vi "Host - TCP - Engine.vi"() -> ()   [LabVIEW 2017]
uses:
  TCP Engine/SubVIs/Read File.ctl
  TCP Engine/Controls/RT- Queue States.ctl
  TCP Engine/TCP/TCP - Signals.ctl
  TCP Engine/TCP/TCP - Signal Names.ctl
  Controls/Control - Testscreen.ctl
  RT/Test Execution/Test - Step Result.ctl
  Controls/Test details.ctl
  TCP Engine/TCP/TCP - Driver Control.ctl
  Variable/Global 1.vi
  TCP Engine/TCP/TCP - Test Settings.ctl
  RT/Controls/RT- Get Set.ctl
panel:
  out "Log Path 2":path
  out "Log Path":path
  out "Waveform Chart":u32(graph)
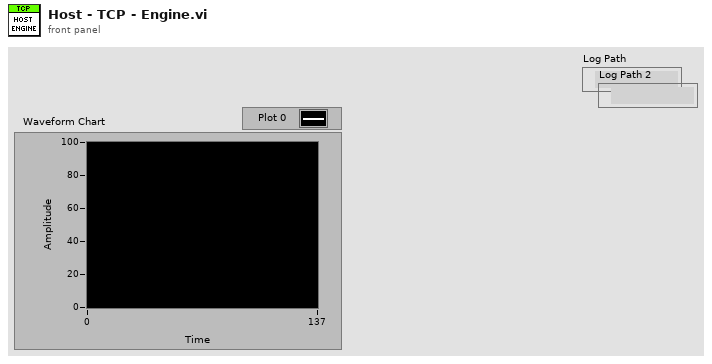
[diagram p1: front panel]
types:
  T1 = typedef "RT- Queue States.ctl" = enum16{"Initialize", "Enqueue", "Enqueue Priority", "Dequeue", "Flush", "Destroy"}
  T2 = typedef "Read File.ctl" = enum16{"Fetch XML", "Open", "Read", "Write", "Close"}
  T3 = typedef "TCP - Test Settings.ctl" = cluster{"Sequence File":string, "Iteration":i32}
  T4 = typedef "TCP - Signals.ctl" = cluster{"Signal":T5, "Value":bool, "Data":variant}
  T5 = typedef "TCP - Signal Names.ctl" = enum16{"Test Running", "Update Sensor Data", "Start Test", "Test Started", "Sequence Complete", "Seuence Aborted", "Abort Test", "Test Settings Updated", "Log Path", "Update Manual Values", "Start Aux Logging", "Aux Log Started", "Stop Aux Logging", "Aux Log Stopped", "Set Dyno Config", "Get PID Values", "Reset Emergency", "Copy Log File", "Download Files", "Send Test Details"}
  T6 = typedef "Control - Testscreen.ctl" = enum16{"No Event", "Init", "Download Files", "Test Running", "Update Test Results", "Machine Unhealthy", "Autotest Started", "Test Aborted", "Sequence Complete", "Update Sensor Data", "Log File Available", "Machine Mode", "Aux Logging Started", "Aux File Saved", "Get PID Values", "View Report", "Exit", "Wait", "Abort", "Copy Log File", "Send Test Details"}
  T7 = typedef "Test - Step Result.ctl" = cluster{"Step Name":string, "Value":dbl, "Success ?":bool, "Stop Seq ?":bool, "Abort":bool, "Sr.No":i32}
  T8 = typedef "RT- Get Set.ctl" = enum16{"Reset", "Get", "Set"}
  T9 = typedef "Test details.ctl" = cluster{"Furnace":string, "Material":string, "Angle":string, "ID":string, "Flowrate":string, "Test Name":string, "Tested By":string}
  T10 = typedef "TCP - Driver Control.ctl" = enum16{"Test Settings", "Boolean Commands", "Test Results", "Send Test Details"}
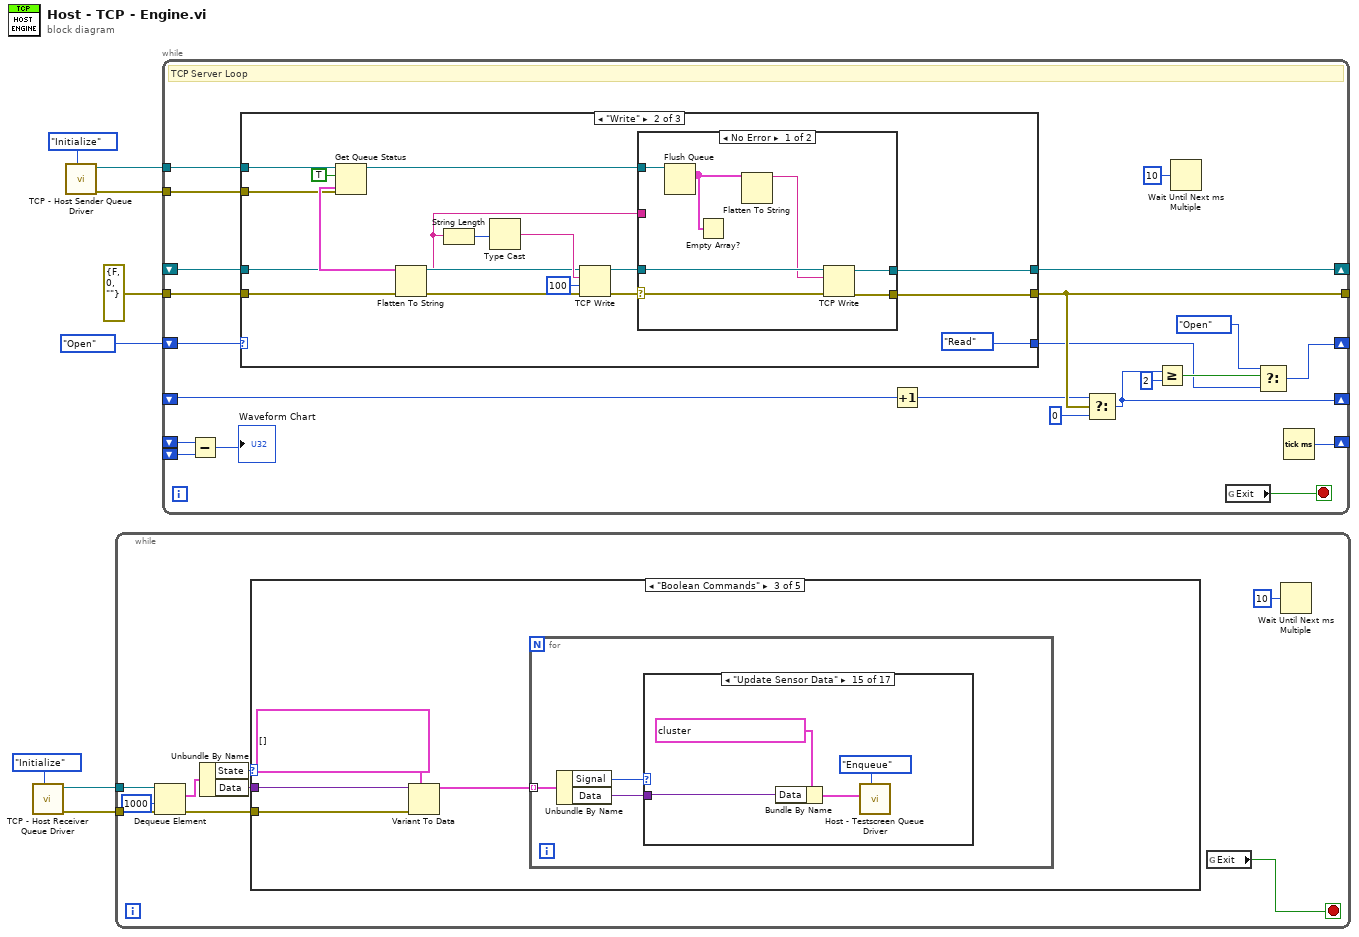
[diagram p0: block diagram]
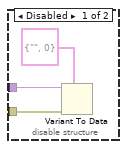
[diagram p3: hidden frame]
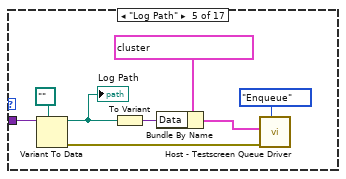
[diagram p9: hidden frame]
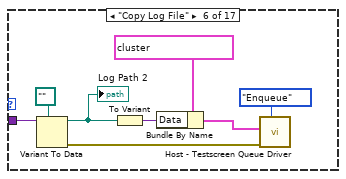
[diagram p10: hidden frame]
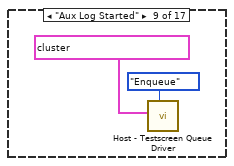
[diagram p13: hidden frame]
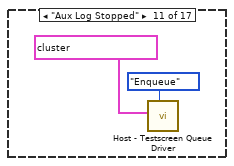
[diagram p15: hidden frame]
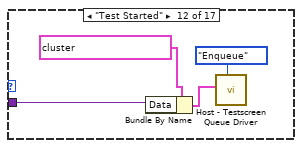
[diagram p16: hidden frame]
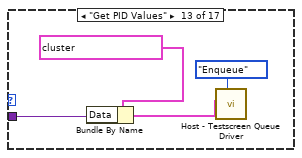
[diagram p17: hidden frame]
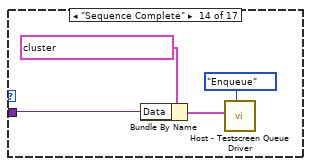
[diagram p18: hidden frame]
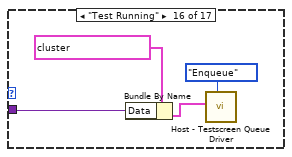
[diagram p19: hidden frame]
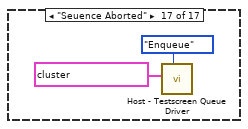
[diagram p20: hidden frame]
diagram:
  n1 = call "TCP - Host Receiver Queue Driver.vi"("Cases"=RT-_Queue_States."Initialize") -> ("error out"=w5:errorcluster, "queue out"=w6:refnum<queue>)  [unwired: 8 in, 1 out]
  n2 = call "TCP - Host Sender Queue Driver.vi"("Cases"=RT-_Queue_States."Initialize") -> ("error out"=w1:errorcluster, "queue out"=w2:refnum<queue>)  [unwired: 8 in, 1 out]
  n3 = while {
    tunnel: w6 -> [w16]
    tunnel: w5 -> [w17]
    stop <- w9 stop-if-true
    n4 = Dequeue Element(queue=w16, timeout in ms (-1)=1000, error in (no error)=w17) -> (element=w14:cluster{"Data":variant, "State":T10}, error out=w15:errorcluster)  [unwired: 2 out]
    n5 = Unbundle By Name(w14) -> ("State"=w12:T10, "Data"=w11:variant)
    n6 = case shown="\"Boolean Commands\"" w12 {
      tunnel: w15 -> [w19 _ w25 w80 w97]
      tunnel: w11 -> [w18 _ w26 w81 w98]
      frame "Test Settings" {
        n7 = disable-structure shown="Enabled" {
          disable-tunnel: w19 -> [w22 _]
          disable-tunnel: w18 -> [w21 _]
          frame Disabled {
            n8 = Variant To Data(error in=w22, type=T3 {"Sequence File"="", "Iteration"=0}, Variant=w21) -> ()  [unwired: 2 out]
          }
          frame Enabled {
          }
        }
      }
      frame Default {
      }
      frame "Boolean Commands" {
        n9 = Variant To Data(error in=w25, type=T4[] [], Variant=w26) -> (data=w23:T4[])  [unwired: 1 out]
        n10 = for {
          tunnel: w23 -> [w29] mode=indexing
          n11 = Unbundle By Name(w29) -> ("Signal"=w28:T5, "Data"=w27:variant)
          n12 = case shown="\"Update Sensor Data\"" w28 {
            tunnel: w27 -> [_ _ _ _ w37 w45 _ _ _ _ _ w52 w55 w60 w64 w68 _]
            frame "Start Test", Default {
            }
            frame "Abort Test" {
            }
            frame "Test Settings Updated" {
            }
            frame "Set Dyno Config" {
            }
            frame "Log Path" {
              n13 = Variant To Data(type=path "", Variant=w37) -> (data=w32:path, error out=w34:errorcluster)  [unwired: 1 in]
              "Log Path" <- w32
              n14 = To Variant(anything=w32) -> (Variant=w31:variant)
              n15 = Bundle By Name(cluster=cluster{"Data":variant, "Enum":T6} {"Data"=variant, "Enum"=enum."Log File Available"} ("Element In"), "Data"=w31) -> (w30:cluster{"Data":variant, "Enum":T6})
              n16 = call "Host - Testscreen Queue Driver.vi"("Cases"=RT-_Queue_States."Enqueue", "error in (no error)"=w34, "Element In"=w30) -> ()  [unwired: 6 in, 3 out]
            }
            frame "Copy Log File" {
              n17 = Variant To Data(type=path "", Variant=w45) -> (data=w40:path, error out=w42:errorcluster)  [unwired: 1 in]
              "Log Path 2" <- w40
              n18 = To Variant(anything=w40) -> (Variant=w39:variant)
              n19 = Bundle By Name(cluster=cluster{"Data":variant, "Enum":T6} {"Data"=variant, "Enum"=enum."Copy Log File"} ("Element In"), "Data"=w39) -> (w38:cluster{"Data":variant, "Enum":T6})
              n20 = call "Host - Testscreen Queue Driver.vi"("Cases"=RT-_Queue_States."Enqueue", "error in (no error)"=w42, "Element In"=w38) -> ()  [unwired: 6 in, 3 out]
            }
            frame "Update Manual Values" {
            }
            frame "Start Aux Logging" {
            }
            frame "Aux Log Started" {
              n21 = call "Host - Testscreen Queue Driver.vi"("Cases"=RT-_Queue_States."Enqueue", "Element In"=cluster{"Data":variant, "Enum":T6} {"Data"=variant, "Enum"=enum."Aux Logging Started"}) -> ()  [unwired: 7 in, 3 out]
            }
            frame "Stop Aux Logging" {
            }
            frame "Aux Log Stopped" {
              n22 = call "Host - Testscreen Queue Driver.vi"("Cases"=RT-_Queue_States."Enqueue", "Element In"=cluster{"Data":variant, "Enum":T6} {"Data"=variant, "Enum"=enum."Aux File Saved"}) -> ()  [unwired: 7 in, 3 out]
            }
            frame "Test Started" {
              n23 = Bundle By Name(cluster=cluster{"Data":variant, "Enum":T6} {"Data"=variant, "Enum"=enum."Autotest Started"} ("Element In"), "Data"=w52) -> (w50:cluster{"Data":variant, "Enum":T6})
              n24 = call "Host - Testscreen Queue Driver.vi"("Cases"=RT-_Queue_States."Enqueue", "Element In"=w50) -> ()  [unwired: 7 in, 3 out]
            }
            frame "Get PID Values" {
              n25 = Bundle By Name(cluster=cluster{"Data":variant, "Enum":T6} {"Data"=variant, "Enum"=enum."Get PID Values"} ("Element In"), "Data"=w55) -> (w54:cluster{"Data":variant, "Enum":T6})
              n26 = call "Host - Testscreen Queue Driver.vi"("Cases"=RT-_Queue_States."Enqueue", "Element In"=w54) -> ()  [unwired: 7 in, 3 out]
            }
            frame "Sequence Complete" {
              n27 = Bundle By Name(cluster=cluster{"Data":variant, "Enum":T6} {"Data"=variant, "Enum"=enum."Sequence Complete"} ("Element In"), "Data"=w60) -> (w58:cluster{"Data":variant, "Enum":T6})
              n28 = call "Host - Testscreen Queue Driver.vi"("Cases"=RT-_Queue_States."Enqueue", "Element In"=w58) -> ()  [unwired: 7 in, 3 out]
            }
            frame "Update Sensor Data" {
              n29 = Bundle By Name(cluster=cluster{"Data":variant, "Enum":T6} {"Data"=variant, "Enum"=enum."Update Sensor Data"} ("Element In"), "Data"=w64) -> (w62:cluster{"Data":variant, "Enum":T6})
              n30 = call "Host - Testscreen Queue Driver.vi"("Cases"=RT-_Queue_States."Enqueue", "Element In"=w62) -> ()  [unwired: 7 in, 3 out]
            }
            frame "Test Running" {
              n31 = Bundle By Name(cluster=cluster{"Data":variant, "Enum":T6} {"Data"=variant, "Enum"=enum."Test Running"} ("Element In"), "Data"=w68) -> (w66:cluster{"Data":variant, "Enum":T6})
              n32 = call "Host - Testscreen Queue Driver.vi"("Cases"=RT-_Queue_States."Enqueue", "Element In"=w66) -> ()  [unwired: 7 in, 3 out]
            }
            frame "Seuence Aborted" {
              n33 = call "Host - Testscreen Queue Driver.vi"("Cases"=RT-_Queue_States."Enqueue", "Element In"=cluster{"Data":variant, "Enum":T6} {"Data"=variant, "Enum"=enum."Test Aborted"}) -> ()  [unwired: 7 in, 3 out]
            }
          }
        }
      }
      frame "Test Results" {
        n34 = Variant To Data(error in=w80, type=T7 {"Step Name"="", "Value"=0.0, "Success ?"=TRUE, "Stop Seq ?"=TRUE, "Abort"=TRUE, "Sr.No"=0} ("element"), Variant=w81) -> (data=w77:T7, error out=w76:errorcluster)
        n35 = disable-structure shown="Enabled" {
          disable-tunnel: w77 -> [w84 w88]
          disable-tunnel: w76 -> [w83 w87]
          disable-tunnel: [w82 w87] -> w75
          disable-tunnel: [_ w86] -> w73
          frame Disabled {
            n36 = call "Test - FGV - Test Results.vi"("Get/Set"=RT-_Get_Set."Set", "error in (no error)"=w83, "Step Result"=w84) -> ("error out"=w82:errorcluster)  [unwired: 7 in, 1 out]
          }
          frame Enabled {
            n37 = To Variant(anything=w88) -> (Variant=w86:variant)
          }
        }
        n38 = Bundle By Name(cluster=cluster{"Data":variant, "Enum":T6} {"Data"=variant, "Enum"=enum."Update Test Results"} ("Element In"), "Data"=w73) -> (w72:cluster{"Data":variant, "Enum":T6})
        n39 = call "Host - Testscreen Queue Driver.vi"("Cases"=RT-_Queue_States."Enqueue", "error in (no error)"=w75, "Element In"=w72) -> ()  [unwired: 6 in, 3 out]
      }
      frame "Send Test Details" {
        (unwired) T7 {"Step Name"="", "Value"=0.0, "Success ?"=TRUE, "Stop Seq ?"=TRUE, "Abort"=TRUE, "Sr.No"=0} ("element")
        n40 = Variant To Data(error in=w97, type=T9 {"Furnace"="Furnace A", "Material"="Coke", "Angle"="Multi Angle", "ID"="Trajectory 9", "Flowrate"="Flow", "Test Name"="Coke Burn", "Tested By"="Anirban"} ("Test details"), Variant=w98) -> (data=w95:T9, error out=w94:errorcluster)
        n41 = disable-structure shown="Enabled" {
          disable-tunnel: w95 -> [w101 w105]
          disable-tunnel: w94 -> [w100 w104]
          disable-tunnel: [w99 w104] -> w93
          disable-tunnel: [_ w103] -> w91
          frame Disabled {
            n42 = call "Test - FGV - Test Results.vi"("Get/Set"=RT-_Get_Set."Set", "error in (no error)"=w100, "Step Result"=w101) -> ("error out"=w99:errorcluster)  [unwired: 7 in, 1 out]
          }
          frame Enabled {
            n43 = To Variant(anything=w105) -> (Variant=w103:variant)
          }
        }
        n44 = Bundle By Name(cluster=cluster{"Data":variant, "Enum":T6} {"Data"=variant, "Enum"=enum."Send Test Details"} ("Element In"), "Data"=w91) -> (w90:cluster{"Data":variant, "Enum":T6})
        n45 = call "Host - Testscreen Queue Driver.vi"("Cases"=RT-_Queue_States."Enqueue", "error in (no error)"=w93, "Element In"=w90) -> ()  [unwired: 6 in, 3 out]
      }
    }
    n46 = global read "Global 1.vi" "Exit"() -> (w9:bool)
    n47 = Wait Until Next ms Multiple(millisecond multiple=u32 10) -> ()  [unwired: 1 out]
  }
  n48 = while {
    shift-right: [w126] -> _
    shift-left: _ -> [w125]
    shift-right: [w116] -> _
    shift-left: Read_File."Open" ("R/W") -> [w127]
    shift-right: [w119] -> _
    shift-left: _ -> [w121]
    tunnel: w2 -> [w114]
    tunnel: w1 -> [w113]
    tunnel: errorcluster {"status"=FALSE, "code"=0, "source"=""} ("error out") -> [w124]
    tunnel: [w123] -> _
    shift-right: [w110] -> _
    shift-left: _ -> [w109]
    shift-left: _ -> [w108]
    stop <- w106 stop-if-true
    # "TCP Server Loop"
    n49 = Subtract(x=w109, y=w108) -> (x-y=→"Waveform Chart":u32)
    n50 = case shown="\"Write\"" w127 {
      tunnel: [w132 w175 w191] -> w126
      tunnel: [w131 w174 w190] -> w123
      tunnel: w125 -> [w137 w163 _]
      tunnel: w124 -> [w136 w166 _]
      tunnel: [Read_File."Write" ("R/W") Read_File."Read" ("R/W") w192] -> w112
      tunnel: w114 -> [_ w168 _]
      tunnel: w113 -> [_ w167 _]
      frame "Read", Default {
        n51 = TCP Read(connection ID=w137, bytes to read=4, error in (no error)=w136, 9:100 ("timeout ms (25000)")) -> (connection ID out=w135:refnum<k5>, data out=w130:string, error out=w128:errorcluster)  [unwired: 1 out]
        n52 = case shown="No Error" w128 {
          selector: w128 -> [w142 w159]
          tunnel: w135 -> [w147 w160]
          tunnel: [w146 w160] -> w132
          tunnel: [w141 w159] -> w131
          tunnel: w130 -> [w144 _]
          frame No Error {
            n53 = Type Cast(type=4 ("bytes to read"), x=w144) -> (*(type *) &x=w143:i32)
            n54 = TCP Read(connection ID=w147, bytes to read=w143, error in (no error)=w142, 9:2000 ("timeout ms (25000)")) -> (connection ID out=w146:refnum<k5>, data out=w140:string, error out=w139:errorcluster)  [unwired: 1 out]
            n55 = case shown="No Error" w139 {
              selector: w139 -> [w150 w158]
              tunnel: w140 -> [w151 _]
              tunnel: [w153 w158] -> w141
              frame No Error {
                n56 = Unflatten From String(type=cluster{"Data":variant, "State":T10}[] [], binary string=w151, error in (no error)=w150) -> (value=w148:cluster{"Data":variant, "State":T10}[], error out=w149:errorcluster)  [unwired: 2 in, 1 out]
                n57 = for {
                  tunnel: w148 -> [w154] mode=indexing
                  shift-right: [w156] -> w153
                  shift-left: w149 -> [w155]
                  n58 = call "TCP - Host Receiver Queue Driver.vi"("Cases"=RT-_Queue_States."Enqueue", "error in (no error)"=w155, "Element In"=w154) -> ("error out"=w156:errorcluster)  [unwired: 6 in, 2 out]
                }
              }
              frame Error {
              }
            }
          }
          frame Error {
          }
        }
      }
      frame "Write" {
        n59 = Get Queue Status(queue=w168, return elements? (F)=TRUE, error in (no error)=w167) -> (queue out=w161:refnum<queue>, elements=w170:cluster{"Data":variant, "State":T10}[])  [unwired: 6 out]
        n60 = Flatten To String(anything=w170, error in (no error)=w166) -> (data string=w162:string, error out=w165:errorcluster)  [unwired: 2 in, 1 out]
        n61 = String Length(string=w162) -> (length=w171:i32)
        n62 = Type Cast(x=w171) -> (*(type *) &x=w164:string)  [unwired: 1 out]
        n63 = TCP Write(connection ID=w163, data in=w164, error in (no error)=w165, 9:100 ("timeout ms (25000)")) -> (connection ID out=w176:refnum<k5>, error out=w172:errorcluster)  [unwired: 1 out]
        n64 = case shown="No Error" w172 {
          selector: w172 -> [w181 w185]
          tunnel: w176 -> [w184 w186]
          tunnel: [w183 w186] -> w175
          tunnel: [w182 w185] -> w174
          tunnel: w162 -> [_ _]
          tunnel: w161 -> [w180 _]
          frame No Error {
            n65 = Flush Queue(queue=w180) -> (remaining elements=w179:cluster{"Data":variant, "State":T10}[])  [unwired: 1 in, 2 out]
            n66 = Empty Array?(array=w179) -> ()  [unwired: 1 out]
            n67 = Flatten To String(anything=w179) -> (data string=w178:string)  [unwired: 3 in, 2 out]
            n68 = TCP Write(connection ID=w184, data in=w178, error in (no error)=w181) -> (connection ID out=w183:refnum<k5>, error out=w182:errorcluster)  [unwired: 2 out]
          }
          frame Error {
          }
        }
      }
      frame "Open" {
        (unwired) "localhost" ("address")
        (unwired) "192.168.0.3" ("address")
        w188 = u16 6340  # port
        w189 = 2000  # timeout (ms)
        n69 = TCP Open Connection(address="169.254.10.138" ("service name"), remote port or service name=w188, timeout ms (60000)=w189) -> (connection ID=w191:refnum<k5>, error out=w190:errorcluster)  [unwired: 2 in]
        n70 = Select(t=Read_File."Open", s=w190, f=Read_File."Read" ("R/W")) -> (s? t:f=w192:T2)
      }
    }
    n71 = Increment(x=w121) -> (x+1=w120:i32)
    n72 = Select(t=w120, s=w123, f=0) -> (s? t:f=w119:i32)
    n73 = Greater Or Equal?(x=w119, y=2) -> (x >= y?=w117:bool)
    n74 = Wait Until Next ms Multiple(millisecond multiple=u32 10) -> ()  [unwired: 1 out]
    n75 = global read "Global 1.vi" "Exit"() -> (w106:bool)
    n76 = Select(t=Read_File."Open" ("f"), s=w117, f=w112) -> (s? t:f=w116:T2)
    n77 = Tick Count (ms)() -> (millisecond timer value=w110:u32)
  }
